vi "Write Parameters.vi"(8 "error in (no error)":errorcluster, 10 "Parameters":T1, 11 "ActiveFrontEndModule configuration in":refnum<class "ActiveFrontEndModule configuration.lvclass">) -> (0 "error out":errorcluster, 3 "ActiveFrontEndModule configuration out":refnum<class "ActiveFrontEndModule configuration.lvclass">)   [LabVIEW 2017, in "ActiveFrontEndModule configuration.lvclass"]
uses:
  ActiveFrontEndModule configuration.lvclass
  <vilib>/NI/PowerElectronicsControl/ActiveFrontEnd/AFE/Parameters.ctl
  <vilib>/NI/PowerElectronicsControl/ActiveFrontEnd/AFE/Mode.ctl
  ActiveFrontEndModule configuration.lvclass/ActiveFrontEndModule configuration.ctl
  <vilib>/NI/PowerElectronicsControl/ActiveFrontEnd/AFE/ActiveFrontEnd.lvlib
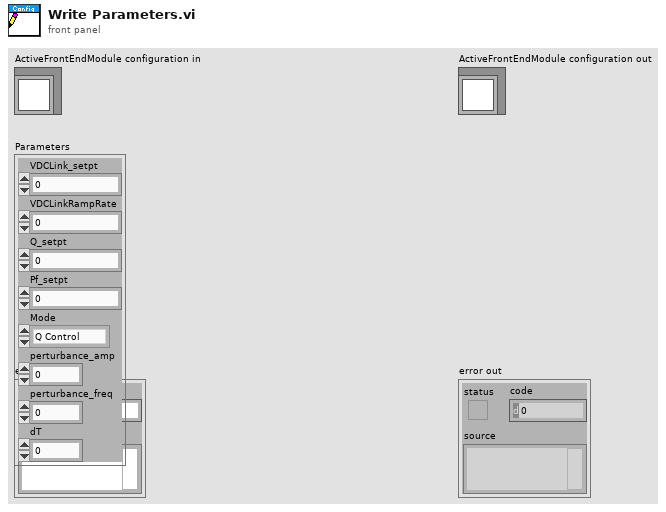
[diagram p1: front panel]
types:
  T1 = typedef "ActiveFrontEnd.lvlib/Parameters.ctl" = cluster{"VDCLink_setpt":sgl, "VDCLinkRampRate":sgl, "Q_setpt":sgl, "Pf_setpt":sgl, "Mode":T2, "perturbance_amp":sgl, "perturbance_freq":sgl, "dT":sgl}
  T2 = typedef "ActiveFrontEnd.lvlib/Mode.ctl" = enum16{"Q Control", "Pf Control"}
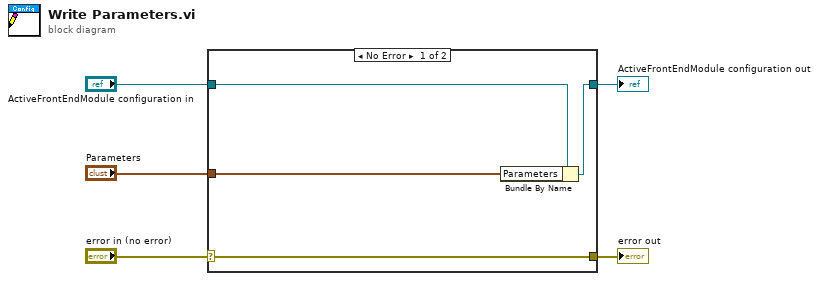
[diagram p0: block diagram]
diagram:
  n1 = case shown="No Error" "error in (no error)" {
    selector: "error in (no error)" -> [w9 w10]
    tunnel: [w9 w10] -> w4
    tunnel: [w7 w11] -> w2
    tunnel: "ActiveFrontEndModule configuration in" -> [w8 w11]
    tunnel: "Parameters" -> [w6 _]
    frame No Error {
      n2 = Bundle By Name(cluster=w8, "Parameters"=w6) -> (w7:refnum<class "ActiveFrontEndModule configuration.lvclass">)
    }
    frame Error {
    }
  }
  "error out" <- w4
  "ActiveFrontEndModule configuration out" <- w2
